vi "Header file compatibility manager.vi"() -> (0 "ROI file format version":i32, 1 "[ROI Time (us)]":dbl[](array[numeric]), 2 "Z-Stack Header data":T1={"Number of POI"=0, "Number of Miniscans"=0, "Number of Trials"=0, "Number of Cycles "=0, "# Averaged Frames"=0, "Laser power (%)"=0, "Pockels"=0.0, "Acquisition Length (sec)"=0.0, "Fill time (us)"=0.0, "DwellTime (us)"=0.0, "Miniscan Dwell time per pixel (us)"=0.0, "PMT 1"=0.0, "PMT 2"=0.0, "Back Apperture"=0.0, "Zoom"=0.0, "Number of Pixels in Miniscan"=0, "Frame Size"=200, "Field of View"=0.0, "X centre"=0.0, "Y centre"=0.0, "AOL Z"=0.0} {"Frame Size" items=["100X100"=100, "128X128"=128, "200X200"=200, "256X256"=256, "512X512"=512, "1024x1024"=1024, "2048x2048"=2048]; "Back Apperture" format="%#.6g"; "Pockels" format="%#.6g"; "PMT 2" format="%#.6g"; "PMT 1" format="%#.6g"; "Miniscan Dwell time per pixel (us)" format="%#.6g"; "Zoom" format="%#.6g"; "DwellTime (us)" format="%#.6g"; "Acquisition Length (sec)" format="%#.6g"; "Fill time (us)" format="%#.6g"}, 3 "[Pixels in ROI]":i32[](array[numeric]))   [LabVIEW 2017]
uses:
  Experiment header interface/Typedefs/Header parameters cluster-Zstack.ctl
  Typedefs/Frame Size.ctl
  Typedefs/Get-Set-Clear Control.ctl
  Experiment header interface/Typedefs/Header file interface module functions enum.ctl
  Global Variables/General Globals.vi
panel:
  # "Zstack header parameters"
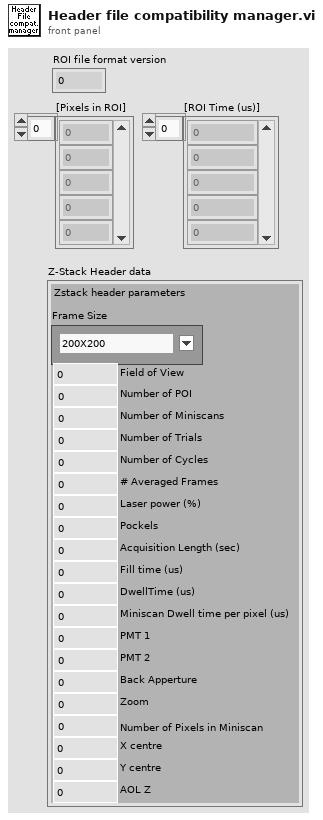
[diagram p1: front panel]
types:
  T1 = typedef "Header parameters cluster-Zstack.ctl" = cluster{"Number of POI":u16, "Number of Miniscans":u16, "Number of Trials":u16, "Number of Cycles ":u16, "# Averaged Frames":u16, "Laser power (%)":u8, "Pockels":dbl, "Acquisition Length (sec)":dbl, "Fill time (us)":dbl, "DwellTime (us)":dbl, "Miniscan Dwell time per pixel (us)":dbl, "PMT 1":dbl, "PMT 2":dbl, "Back Apperture":dbl, "Zoom":dbl, "Number of Pixels in Miniscan":u16, "Frame Size":T2, "Field of View":dbl, "X centre":dbl, "Y centre":dbl, "AOL Z":dbl}
  T2 = typedef "Frame Size.ctl" = u16
  T3 = typedef "Header file interface module functions enum.ctl" = enum16{"Load experiment header file", "Save experiment header file", "Clear stored values", "Read stored values", "Update specific value in memory", "Update values in memory"}
  T4 = typedef "Get-Set-Clear Control.ctl" = enum16{"Get", "Set", "Clear"}
  T5 = typedef "Functional Parameters Cluster.ctl" = cluster{"ROI data":dbl[][], "ROI format version":i32, "Norm ROI data":dbl[][], "Norm. ROI format version":i32, "Z norm":dbl[], "Z norm format version":i32}
  T6 = typedef "Header parameters cluster-ALL.ctl" = cluster{"LOGIN":T7, "GLOBAL PARAMETERS":T8, "IMAGING MODES":T10, "TIME SERIES":T11, "MOTOR Z-STACK ":T13, "AOL Z-STACK":T14, "FUNCTIONAL IMAGING":T15, "MOVEMENT CORRECTION":T16, "CALIBRATION":T18, "STATISTICS":T19, "BIOLOGY INFORMATION":T20}
  T7 = typedef "Header params -Login.ctl" = cluster{"User":string, "Profile":string, "Software Version":string, "Experiment Date Time":timestamp}
  T8 = typedef "Header params-Global Parameters.ctl" = cluster{"MicroscopeID":string, "Microscope Type":string, "Objective":string, "Field of View (um)":dbl, "Fill time (us)":dbl, "Experiment Type":T9, "Stimuli Trigger":bool, "Speed Logging":bool}
  T9 = typedef "Experiment Type.ctl" = enum16{"In vivo", "In vitro", "Testing", "Calibration", "Other"}
  T10 = typedef "Header params-Imaging Modes.ctl" = cluster{"Time Series":bool, "Motor Zstack":bool, "AOL Zstack":bool, "Functional Imaging":bool}
  T11 = typedef "Header params-Time Series.ctl" = cluster{"Basic Image meta data":T12, "AOL z":dbl}
  T12 = typedef "Header params-Basic image meta data.ctl" = cluster{"Wavelength (nm)":dbl, "# averaged frames":dbl, "laser power (%)":dbl, "Pockels":dbl, "pixel dwell time (us)":dbl, "pmt 1":dbl, "pmt 2":dbl, "back apperture":dbl, "zoom":dbl, "field of view":dbl, "frame size":dbl, "AOL x centre":dbl, "AOL y centre":dbl, "Stage x position":dbl, "Stage y position":dbl, "Stage z position":dbl}
  T13 = typedef "Header params-Motor Z-stack.ctl" = cluster{"Hdr Basic Image meta data":T12, "Z Start":dbl, "Z Stop":dbl, "No of Planes":dbl}
  T14 = typedef "Header params-AOL Z-stack.ctl" = cluster{"Hdr Basic Image meta data":T12, "Z Start":dbl, "Z Stop":dbl, "No of Planes":dbl}
  T15 = typedef "Header params-Functional Imaging.ctl" = cluster{"Functional Mode":enum16{"Point", "Line", "Patch", "Plane", "Volume"}, "Pockels Modulation":bool, "Number of pois":dbl, "Number of miniscans":dbl, "Number of cycles":dbl, "Number of trials":dbl, "Miniscan dwell time per pixel (us)":dbl, "Number of pixels in miniscan":dbl, "poi dwell time":dbl, "Rectangle ROI length":dbl, "Rectangle ROI height":dbl, "AOL mode":dbl, "Plane mode":dbl, "video length (sec)":dbl, "Frame rate (fps)":dbl, "Stimuli Timing (usec)":dbl, "Acquisition Length":dbl, "Basic Image meta data":T12, "Z Start (um)":dbl, "Z Stop (um)":dbl}
  T16 = typedef "Header params-Movement correction.ctl" = cluster{"Movement Correction":bool, "Axial Reference":bool, "Reference Size":dbl, "Reference Source":T17, "Reference dwell time (us)":dbl, "Number of Z lines":dbl, "Size of Z pixels":dbl, "Axial Pixels":dbl, "Reference Zoom":dbl, "Reference Average":dbl, "Proportional Scale":dbl, "Integral Scale":dbl, "Proportional Scale Z":dbl, "Integral Scale Z":dbl, "Scan Interval":dbl, "Ref Plot Refresh Rate":dbl}
  T17 = typedef "Reference source.ctl" = enum16{"Green channel", "Red channel"}
  T18 = typedef "Header params-Calibration Setup.ctl" = cluster{"Pockels Calibration File":path, "Calibration_ini file":path, "Setup_ini file":path}
  T19 = typedef "Header params-statistics.ctl" = cluster{"Z-stack duration (sec)":dbl, "Number of acquired data-points":dbl, "Acquisition time (ms)":dbl, "Number of acquired frames":dbl}
  T20 = typedef "Biology Information.ctl" = cluster{"Animal Code or Name":string, "Animal DoB":string, "Animal Age":string, "Animal Sex":string, "Animal Weight":string, "Date of Injection":string, "Date of Implant":string, "Site of Injection":string, "Animal Ear Notch":string, "AAV constructs":string, "Genetic background":string, "Optical reporter":string, "Region of brain imaged":string, "Other \ncomments":string}
  T21 = typedef "ROI file columns mapping.ctl" = cluster{"\"ROI index\" column index":i32, "\"ROI ID\" column index":i32, "\"ROI Time (ns)\" column index":i32, "\"Pixels in ROI\" column index":i32, "\"X (X start)\" column index":i32, "\"Y (Y start)\" column index":i32, "\"Z (Z start)\" column index":i32, "\"X (X stop)\" column index":i32, "\"Y (Y stop)\" column index":i32, "\"Z (Z stop)\" column index":i32, "\"Angle (deg)\" column index":i32, "Composite ID":i32, "Number of lines":i32, "Frame Size":i32, "Zoom":i32, "Laser Power (%)":i32, "ROI group ID":i32}
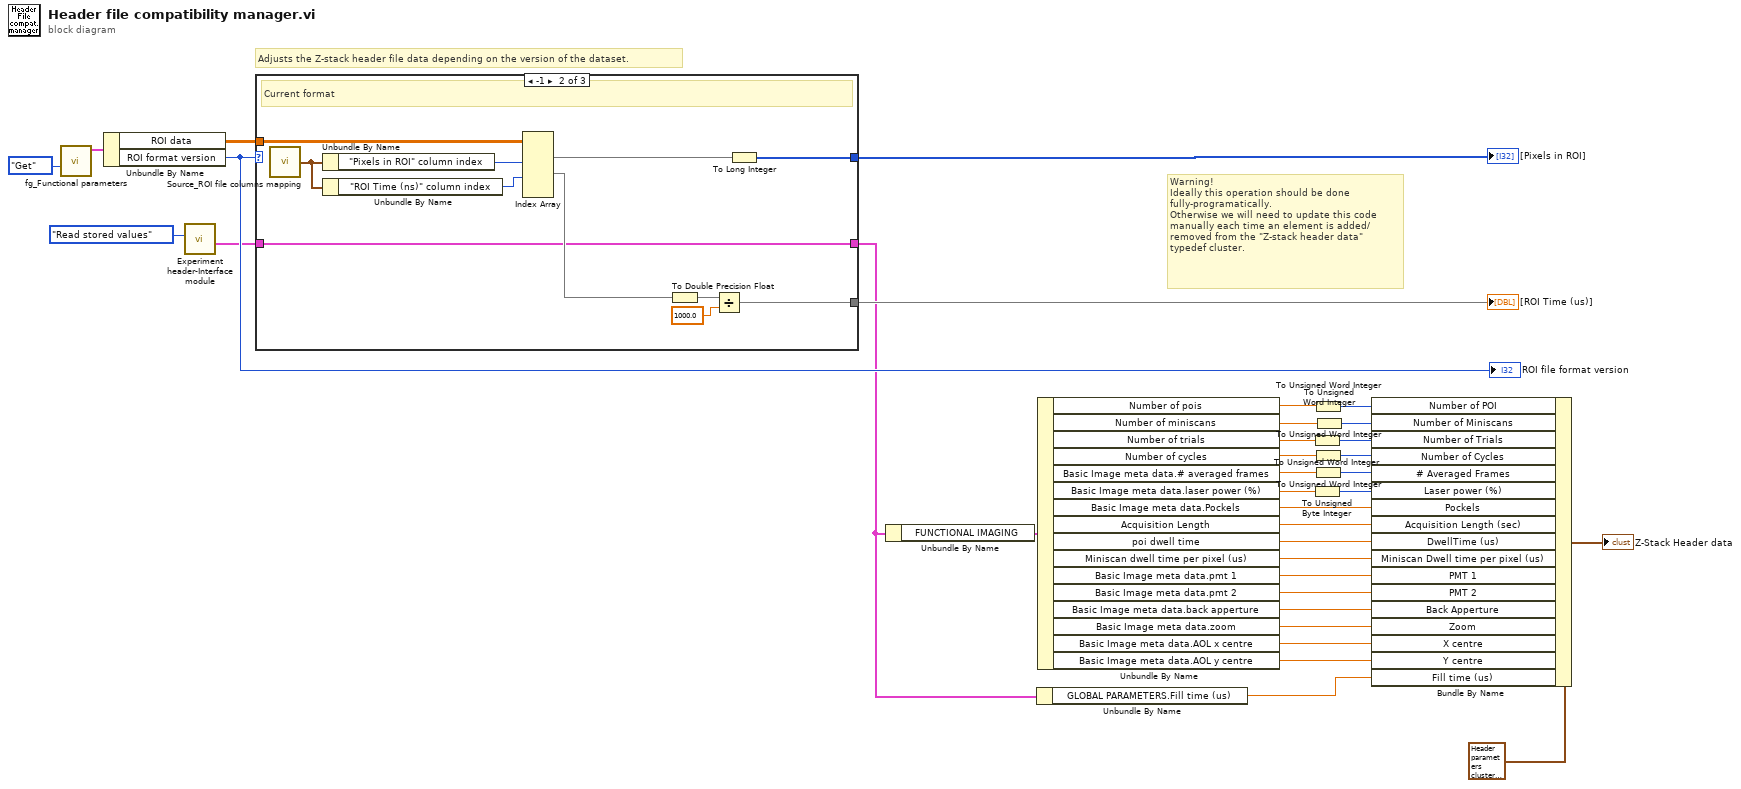
[diagram p0: block diagram]
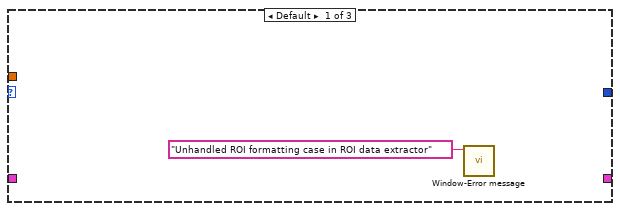
[diagram p2: hidden frame]
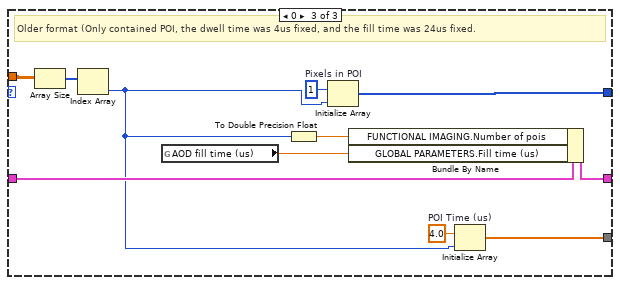
[diagram p3: hidden frame]
diagram:
  # "Warning!\nIdeally this operation should be done fully-programatically.\nOtherwise we will need to update this code manually each time an element is added/removed from the \"Z-stack header data\" typedef cluster."
  # "Adjusts the Z-stack header file data depending on the version of the dataset."
  n1 = call "fg_Functional parameters.vi"("Function"=Get-Set-Clear_Control."Get") -> ("Functional Parameters"=w31:T5)  [unwired: 7 in, 3 out]
  n2 = Unbundle By Name(w31) -> ("ROI data"=w33:dbl[][], "ROI format version"=w30:i32)
  "ROI file format version" <- w30
  n3 = call "Experiment header-Interface module.vi"("Function"=Header_file_interface_module_functions_enum."Read stored values") -> ("All header parameters out"=w28:T6)  [unwired: 9 in, 1 out]
  n4 = case shown="-1" w30 {
    tunnel: w33 -> [_ w46 w58]
    tunnel: [_ w44 w53] -> w34
    tunnel: [_ w38 w55] -> w35
    tunnel: [_ w37 w50] -> w2
    tunnel: w28 -> [_ w37 w52]
    frame Default {
      n5 = call "Window-Error message.vi"("Message"="Unhandled ROI formatting case in ROI data extractor" ("message")) -> ()  [unwired: 10 in, 1 out]
    }
    frame -1 {
      # "Current format"
      n6 = call "Source_ROI file columns mapping.vi"() -> ("ROI file columns mapping"=w39:T21)  [unwired: 1 in]
      n7 = Unbundle By Name(w39) -> ("\"Pixels in ROI\" column index"=w45:i32)
      n8 = Unbundle By Name(w39) -> ("\"ROI Time (ns)\" column index"=w43:i32)
      n9 = Index Array(array=w46, index (col) #1=w45, index (col) #2=w43) -> (element #1=w47:dbl[], element #2=w40:dbl[])  [unwired: 4 in, 1 out]
      n10 = To Double Precision Float(number=w40) -> (double precision float=w41:dbl[])
      n11 = Divide(x=w41, y=1000.0) -> (x/y=w38:dbl[])
      n12 = To Long Integer(number=w47) -> (32bit integer=w44:i32[])
    }
    frame 0 {
      w54 = 1  # Pixels in POI
      w56 = 4.0  # POI Time (us)
      # "Older format (Only contained POI, the dwell time was 4us fixed, and the fill time was 24us fixed."
      n13 = Array Size(array=w58) -> (size(s)=w57:i32[])
      n14 = Index Array(array=w57) -> (element=w48:i32)  [unwired: 1 in]
      n15 = global read "General Globals.vi" "AOD fill time (us)"() -> (w51:dbl)
      n16 = To Double Precision Float(number=w48) -> (double precision float=w49:dbl)
      n17 = Initialize Array(w54, w48) -> (w53:i32[])
      n18 = Bundle By Name(cluster=w52, "FUNCTIONAL IMAGING.Number of pois"=w49, "GLOBAL PARAMETERS.Fill time (us)"=w51) -> (w50:T6)
      n19 = Initialize Array(w56, w48) -> (w55:dbl[])
    }
  }
  "[ROI Time (us)]" <- w35
  "[Pixels in ROI]" <- w34
  n20 = Unbundle By Name(w2) -> ("FUNCTIONAL IMAGING"=w15:T15)
  n21 = Unbundle By Name(w2) -> ("GLOBAL PARAMETERS.Fill time (us)"=w1:dbl)
  n22 = Unbundle By Name(w15) -> ("Number of pois"=w14:dbl, "Number of miniscans"=w12:dbl, "Number of trials"=w11:dbl, "Number of cycles"=w10:dbl, "Basic Image meta data.# averaged frames"=w9:dbl, "Basic Image meta data.laser power (%)"=w8:dbl, "Basic Image meta data.Pockels"=w26:dbl, "Acquisition Length"=w25:dbl, "poi dwell time"=w24:dbl, "Miniscan dwell time per pixel (us)"=w23:dbl, "Basic Image meta data.pmt 1"=w22:dbl, "Basic Image meta data.pmt 2"=w21:dbl, "Basic Image meta data.back apperture"=w20:dbl, "Basic Image meta data.zoom"=w19:dbl, "Basic Image meta data.AOL x centre"=w17:dbl, "Basic Image meta data.AOL y centre"=w16:dbl)
  n23 = To Unsigned Word Integer(number=w11) -> (unsigned 16bit integer=w6:u16)
  n24 = To Unsigned Byte Integer(number=w8) -> (unsigned 8bit integer=w3:u8)
  n25 = To Unsigned Word Integer(number=w14) -> (unsigned 16bit integer=w13:u16)
  n26 = To Unsigned Word Integer(number=w10) -> (unsigned 16bit integer=w5:u16)
  n27 = To Unsigned Word Integer(number=w9) -> (unsigned 16bit integer=w4:u16)
  n28 = To Unsigned Word Integer(number=w12) -> (unsigned 16bit integer=w7:u16)
  n29 = Bundle By Name(cluster=T1 {"Number of POI"=0, "Number of Miniscans"=0, "Number of Trials"=0, "Number of Cycles "=0, "# Averaged Frames"=0, "Laser power (%)"=0, "Pockels"=0.0, "Acquisition Length (sec)"=0.0, "Fill time (us)"=0.0, "DwellTime (us)"=0.0, "Miniscan Dwell time per pixel (us)"=0.0, "PMT 1"=0.0, "PMT 2"=0.0, "Back Apperture"=0.0, "Zoom"=0.0, "Number of Pixels in Miniscan"=0, "Frame Size"=0, "Field of View"=0.0, "X centre"=0.0, "Y centre"=0.0, "AOL Z"=0.0} ("Z-Stack Header data"), "Number of POI"=w13, "Number of Miniscans"=w7, "Number of Trials"=w6, "Number of Cycles"=w5, "# Averaged Frames"=w4, "Laser power (%)"=w3, "Pockels"=w26, "Acquisition Length (sec)"=w25, "DwellTime (us)"=w24, "Miniscan Dwell time per pixel (us)"=w23, "PMT 1"=w22, "PMT 2"=w21, "Back Apperture"=w20, "Zoom"=w19, "X centre"=w17, "Y centre"=w16, "Fill time (us)"=w1) -> (→"Z-Stack Header data":T1)
